vi "Motor EQ.vi"(9 "RIght Input":dbl, 10 "Left Input":dbl, 11 "EQ":dbl) -> (1 "Right Output":dbl, 2 "Left Output":dbl)   [LabVIEW 2013]
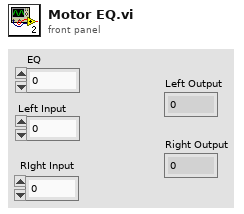
[diagram p1: front panel]
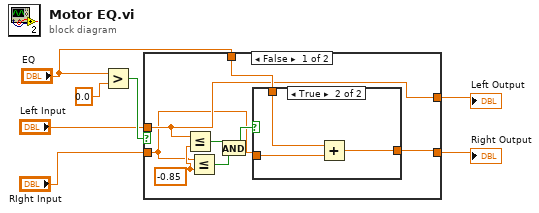
[diagram p0: block diagram]
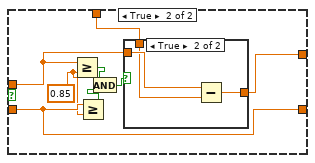
[diagram p3: hidden frame]
diagram:
  n1 = Greater?(x="EQ", y=0.0) -> (0:w6:bool)
  n2 = case shown="False" w6 {
    tunnel: [w9 w27] -> w5
    tunnel: [w14 w23] -> w4
    tunnel: "RIght Input" -> [w8 w23]
    tunnel: "Left Input" -> [w9 w20]
    tunnel: "EQ" -> [w15 w26]
    frame False {
      w10 = -0.85 ("y")
      n3 = Less Or Equal?(x=w9, y=w10) -> (x <= y?=w12:bool)
      n4 = Less Or Equal?(x=w8, y=w10) -> (x <= y?=w11:bool)
      n5 = And(x=w12, y=w11) -> (x .and. y?=w13:bool)
      n6 = case shown="True" w13 {
        tunnel: w15 -> [_ w19]
        tunnel: w8 -> [w16 w18]
        tunnel: [w16 w17] -> w14
        frame False {
        }
        frame True {
          n7 = Add(x=w19, y=w18) -> (x+y=w17:dbl)
        }
      }
    }
    frame True {
      w22 = 0.85 ("y")
      n8 = Greater Or Equal?(x=w20, y=w22) -> (x >= y?=w24:bool)
      n9 = Greater Or Equal?(x=w23, y=w22) -> (x >= y?=w21:bool)
      n10 = And(x=w24, y=w21) -> (x .and. y?=w25:bool)
      n11 = case shown="True" w25 {
        tunnel: [w28 w31] -> w27
        tunnel: w20 -> [w28 w30]
        tunnel: w26 -> [_ w29]
        frame False {
        }
        frame True {
          n12 = Subtract(x=w30, y=w29) -> (x-y=w31:dbl)
        }
      }
    }
  }
  "Left Output" <- w5
  "Right Output" <- w4
